vi "CreateAccessors.vi"(8 "error in (no error)":errorcluster, 11 "GenLVOOP in":refnum<class "GenLVOOP.lvclass">) -> (0 "error out":errorcluster, 3 "GenLVOOP out":refnum<class "GenLVOOP.lvclass">)   [LabVIEW 2013, in "GenLVOOP.lvclass"]
uses:
  GenLVOOP.lvclass
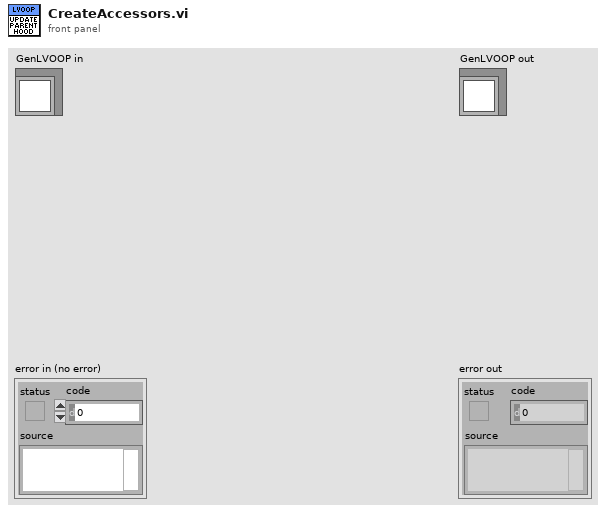
[diagram p1: front panel]
types:
  T1 = typedef "baseClass.lvclass/propertyDef.ctl" = cluster{"Name":string, "types":T2, "UserDefined":string, "Array":bool}
  T2 = typedef "baseClass.lvclass/types.ctl" = enum16{"string", "int", "decimal", "bool", "class", "enum"}
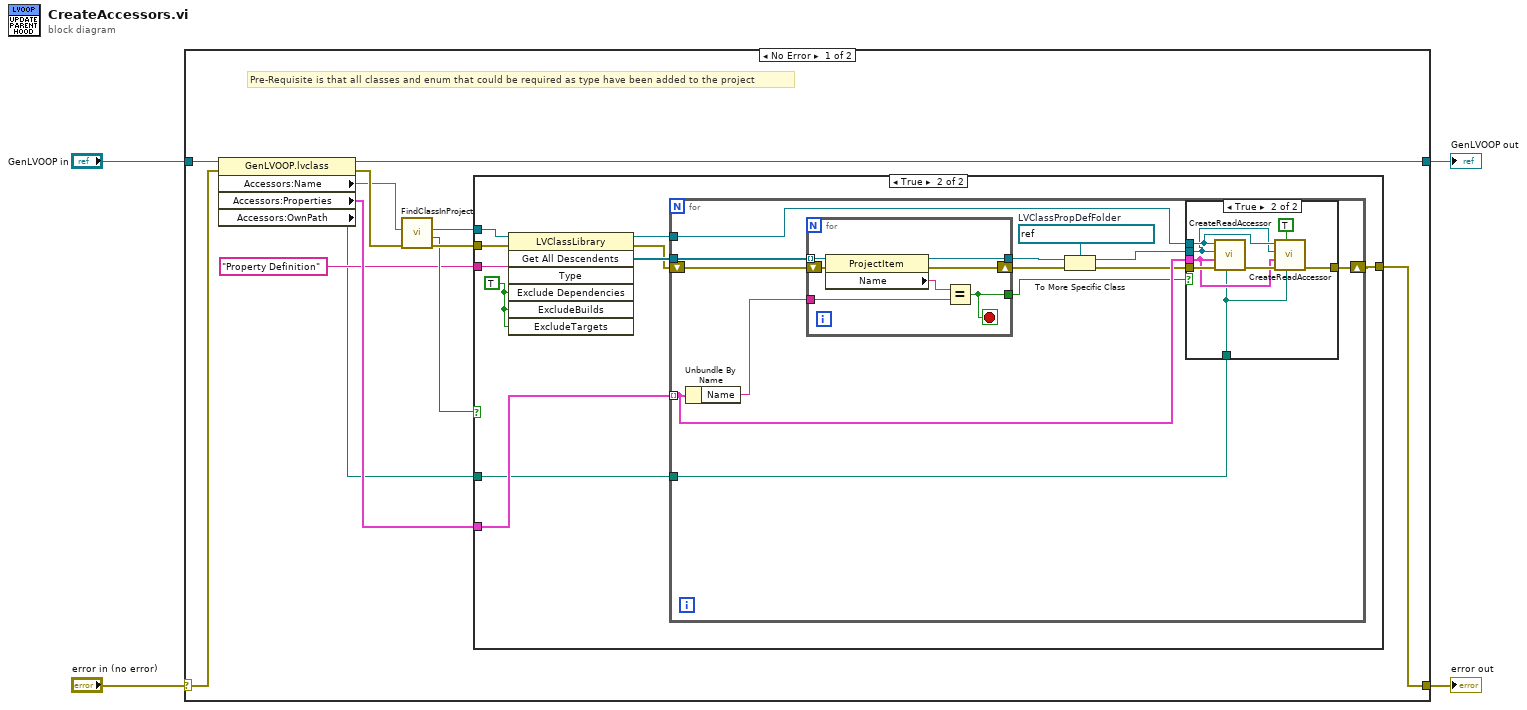
[diagram p0: block diagram]
diagram:
  n1 = case shown="No Error" "error in (no error)" {
    selector: "error in (no error)" -> [w14 w58]
    tunnel: [w15 w58] -> w3
    tunnel: [w10 w57] -> w1
    tunnel: "GenLVOOP in" -> [w16 w57]
    frame No Error {
      # "Pre-Requisite is that all classes and enum that could be required as type have been added to the project"
      n2 = property class="GenLVOOP.lvclass"(reference=w16, error in=w14) -> (reference out=w10:refnum<class "GenLVOOP.lvclass">, error out=w12:errorcluster, "Accessors:Name"=w8:string, "Accessors:Properties"=w9:T1[], "Accessors:OwnPath"=w5:path)
      n3 = call "FindClassInProject.vi"("error in (no error)"=w12, "Name"=w8) -> ("error out"=w11:errorcluster, "Found"=w7:bool, "LVClassLibrary Refnum"=w13:refnum<vi>)  [unwired: 7 in]
      n4 = case shown="True" w7 {
        tunnel: [w17 w21] -> w15
        tunnel: w13 -> [_ w27]
        tunnel: w11 -> [w17 w24]
        tunnel: w9 -> [_ w22]
        tunnel: "Property Definition" ("Type") -> [_ w26]
        tunnel: w5 -> [_ w18]
        frame False {
        }
        frame True {
          w25 = TRUE ("ExcludeDependencies")
          n5 = invoke class="LVClassLibrary" method="Get All Descendents"(reference=w27, error in=w24, "Type"=w26, "Exclude Dependencies"=w25, "ExcludeBuilds"=w25, "ExcludeTargets"=w25) -> (reference out=w19:refnum<vi>, error out=w20:errorcluster, "All Descendents"=w23:refnum<vi>[])  [unwired: 1 in, 4 out]
          n6 = for {
            tunnel: w23 -> [w40]
            tunnel: w22 -> [w32] mode=indexing
            shift-right: [w30] -> w21
            shift-left: w20 -> [w36]
            tunnel: w19 -> [w34]
            tunnel: w18 -> [w28]
            w39 = refnum<vi> refnum  # LVClassPropDefFolder
            n7 = Unbundle By Name(w32) -> ("Name"=w35:string)
            n8 = for {
              tunnel: w40 -> [w56] mode=indexing
              shift-right: [w54] -> w37
              shift-left: w36 -> [w55]
              tunnel: w35 -> [w52]
              tunnel: [w51] -> w38
              tunnel: [w50] -> w29
              stop <- w50 stop-if-true
              n9 = property class="ProjectItem"(reference=w56, error in=w55) -> (reference out=w51:refnum<vi>, error out=w54:errorcluster, "Name"=w53:string)
              n10 = Equal?(x=w53, y=w52) -> (x = y?=w50:bool)
            }
            n11 = To More Specific Class(target class=w39, reference=w38, error in=w37) -> (specific class reference=w33:refnum<vi>, error out=w31:errorcluster)
            n12 = case shown="True" w29 {
              tunnel: w34 -> [_ w46]
              tunnel: w33 -> [_ w45]
              tunnel: w32 -> [_ w44]
              tunnel: w31 -> [w41 w49]
              tunnel: [w41 w47] -> w30
              tunnel: w28 -> [_ w42]
              frame False {
              }
              frame True {
                n13 = call "CreateReadAccessor.vi"("ClassPath"=w42, "error in (no error)"=w49, "properties"=w44, "PropDefFolder"=w45, "LVClassLibrary Refnum"=w46) -> ("error out"=w48:errorcluster)  [unwired: 6 in]
                n14 = call "CreateReadAccessor.vi"("ClassPath"=w42, "Write"=TRUE, "error in (no error)"=w48, "properties"=w44, "PropDefFolder"=w45, "LVClassLibrary Refnum"=w46) -> ("error out"=w47:errorcluster)  [unwired: 5 in]
              }
            }
          }
        }
      }
    }
    frame Error {
    }
  }
  "error out" <- w3
  "GenLVOOP out" <- w1
